vi "全局 总磷.vi"() -> ()   [LabVIEW 2016]
panel:
  in  "总磷":string[][](array[string])
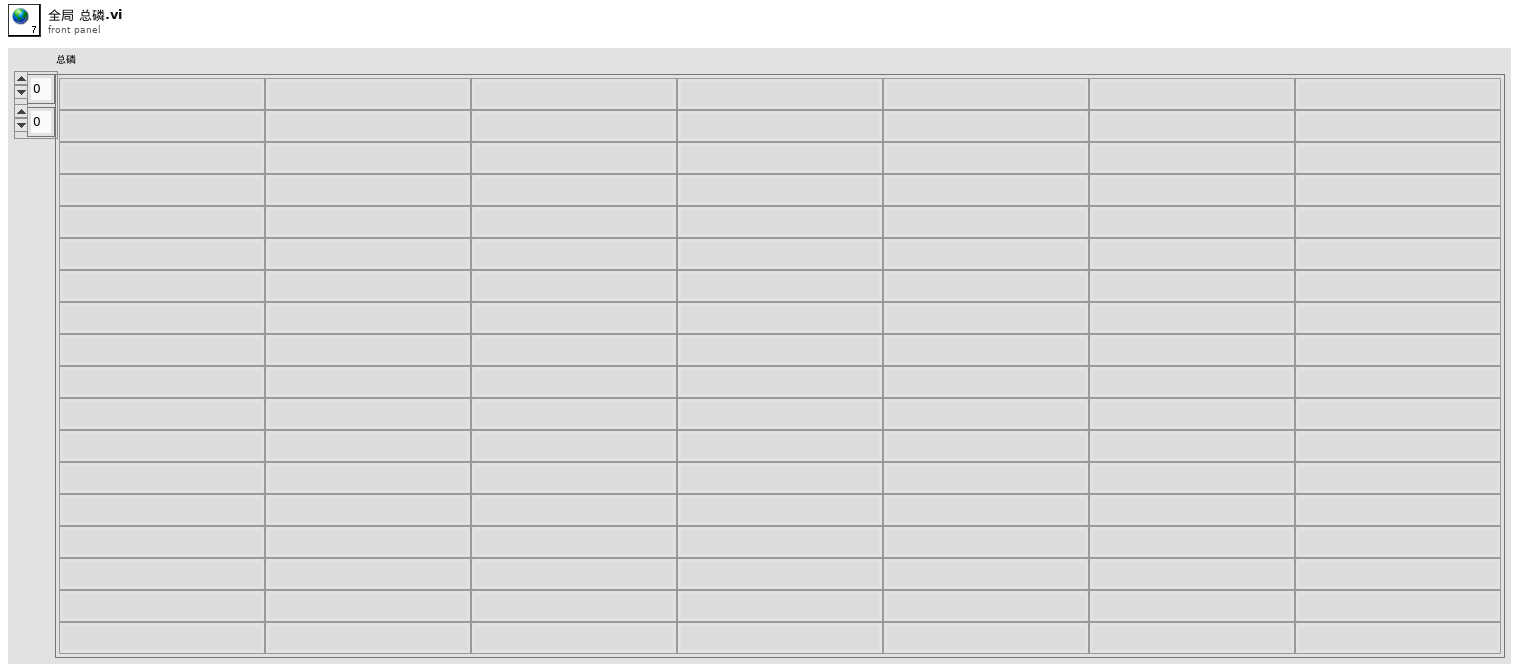
[diagram p1: front panel]
diagram:
